vi "FTW-Publisher-Worker.vi"(1 "keep most recent":i32=1, 2 "Timeout":i32=-1 format="%0d msec", 3 "Endpoint":refnum<class "FTW-Endpoint.lvclass">, 4 "FTW Publisher":refnum<class "FTW-Publisher.lvclass">) -> ()   [LabVIEW 2013, in "FTW-Publisher.lvclass"]
uses:
  FTW-Publisher.lvclass
  Endpoint/FTW-Endpoint.lvclass
  FTW-Publisher.lvclass/FTW-Publisher.ctl
  Message/Base/FTW-Message.lvclass
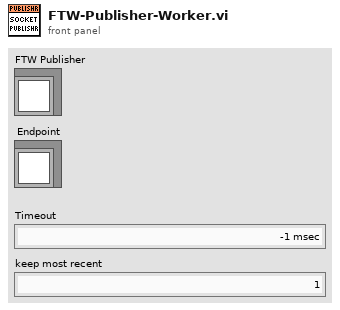
[diagram p1: front panel]
types:
  T1 = cluster{"Message":refnum<user-event>, "Shutdown":refnum<user-event>}
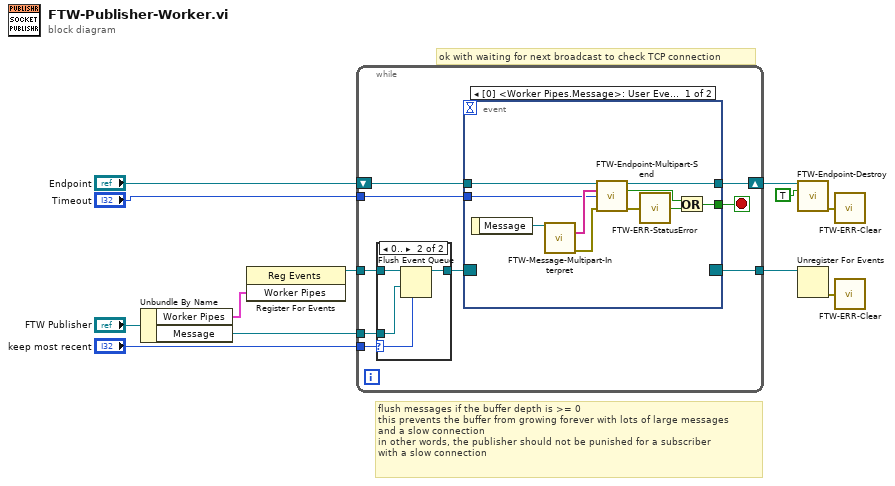
[diagram p0: block diagram]
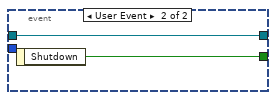
[diagram p3: hidden frame]
diagram:
  # "flush messages if the buffer depth is >= 0\nthis prevents the buffer from growing forever with lots of large messages\nand a slow connection\nin other words, the publisher should not be punished for a subscriber\nwith a slow connection"
  # "ok with waiting for next broadcast to check TCP connection"
  n1 = Unbundle By Name("FTW Publisher") -> ("Worker Pipes"=w2:T1, "Message"=w3:refnum<user-event>)
  n2 = register-events(w2) -> (reference out=w9:refnum<event-registration>)  [unwired: 2 in, 1 out]
  n3 = while {
    tunnel: w9 -> [w21]
    tunnel: [w18] -> w11
    shift-right: [w17] -> w12
    shift-left: "Endpoint" -> [w20]
    tunnel: "Timeout" -> [w15]
    tunnel: "keep most recent" -> [w14]
    tunnel: w3 -> [w13]
    stop <- w19 stop-if-true
    n4 = case shown="0.." w14 {
      selector: w14 -> [_ w24]
      tunnel: w21 -> [w22 w26]
      tunnel: [w22 w25] -> w16
      tunnel: w13 -> [_ w23]
      frame ..-1 {
      }
      frame 0.. {
        n5 = Flush Event Queue(0:w26, 2:w23, 5:w24) -> (8:w25:refnum<event-registration>)  [unwired: 3 in, 2 out]
      }
    }
    n6 = event shown="[0] <Worker Pipes.Message>: User Event" {
      selector: w16 -> [_ _]
      dyn-events: [_ _] -> w18
      timeout: _ -> [_ _]
      tunnel: w20 -> [w36 w38]
      tunnel: [w29 w37] -> w19
      tunnel: [w35 w38] -> w17
      tunnel: w15 -> [w27 _]
      event User Event {
        n7 = event-data() -> ("Message"=w33:refnum<class "FTW-Message.lvclass">)  [unwired: 1 in]
        n8 = call-dynamic "FTW-Message-Multipart-Interpret.vi"("FTW Message"=w33) -> ("Message Parts"=w30:string[], "error out"=w31:errorcluster)  [unwired: 12 in, 1 out]
        n9 = call-dynamic "FTW-Endpoint-Multipart-Send.vi"("FTW Endpoint"=w36, "Multipart Message"=w30, "Timeout"=w27, "error in"=w31) -> ("FTW Endpoint out"=w35:refnum<class "FTW-Endpoint.lvclass">, "Timed out?"=w28:bool, "error out"=w32:errorcluster)  [unwired: 9 in]
        n10 = call "FTW-ERR-StatusError.vi"("error to check"=w32) -> ("Error?"=w34:bool)
        n11 = Or(x=w28, y=w34) -> (x .or. y?=w29:bool)
      }
      event User Event {
        n12 = event-data() -> ("Shutdown"=w37:bool)  [unwired: 1 in]
      }
    }
  }
  n13 = call-dynamic "FTW-Endpoint-Destroy.vi"("FTW Endpoint"=w12, "Force Destroy"=TRUE) -> ("error out"=w7:errorcluster)  [unwired: 13 in]
  n14 = Unregister For Events(event registration refnum=w11) -> (error out=w6:errorcluster)  [unwired: 1 in]
  n15 = call "FTW-ERR-Clear.vi"("error to snuff"=w7) -> ()  [unwired: 1 out]
  n16 = call "FTW-ERR-Clear.vi"("error to snuff"=w6) -> ()  [unwired: 1 out]
